vi "System Editor.vi"() -> ()   [LabVIEW 2013]
uses:
  <vilib>/Utility/miscctls.llb/LVBoundsTypeDef.ctl
  CRYCustom and Run Seq.llb/CRYCustom Cluster.ctl
  CRYCustom and Run Seq.llb/CRYProject Editor Global.vi
  CRYCustom and Run Seq.llb/CRYStepSetup Global.vi
  CRYCustom and Run Seq.llb/CRYMainGlobal.vi
  CRYCustom and Run Seq.llb/CRYMain Sub Window Global.vi
panel:
  out "Custom":string
  out "Custom Bk":string
  in  "AddStep":bool
  in  "Add Lib":bool
  in  "stop":bool
  in  "Load Test":bool
  out "EndFlag":bool
  out "Proper VI No":i32
  in  "Save As":bool
  in  "Load":bool
  in  "Revert":bool
  out "VIMiniumBound":T1
  in  "Board Tab":enum32{"Page 1"}(tab) caption="Control Tab"
  in  "Cancel":bool caption="Apply"
  in  "OK":bool caption="Apply"
  in  "Sub Board Tab":enum32{"Setting", "Help"}(tab)
  in  "Wait for completion":bool
  in  "Working Directory":path
  in  "Command Line":string
  in  "Help":string
  # "Reminder:  You must edit this custom step from\nwithin a sequence for it to remember your settings."
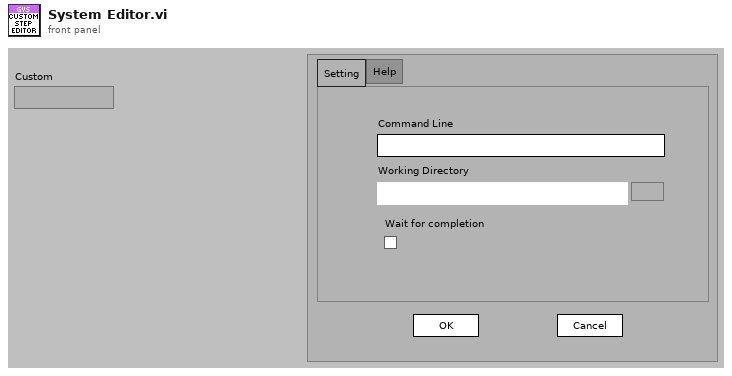
[diagram p1: front panel]
types:
  T1 = typedef "LVBoundsTypeDef.ctl" = cluster{"Width":u32, "Height":u32}
  T2 = cluster{"Command Line":string, "Working Directory":path, "Wait for completion":bool}
  T3 = typedef "CRYStep.ctl" = cluster{"No.VI":i32, "Category":string, "StepName":string, "Seq setup flattened":string, "Comment":string, "Steps config.":bool[], "Jump config":i32[], "Start":dbl, "Increment":dbl, "Name":string, "Unit":string, "Y data":u16, "Y prefix":string, "Y dB ref":dbl, "Y unit":string, "Repeat State Array":cluster{"Start":dbl, "Increment":dbl, "Count":i32, "Num":i32}[]}
  T4 = typedef "CRYCustom Cluster.ctl" = cluster{"Help":string, "Flatten Data":string}
  T5 = cluster{"Load Test":bool, "Add Lib":bool, "OK":bool, "Cancel":bool}
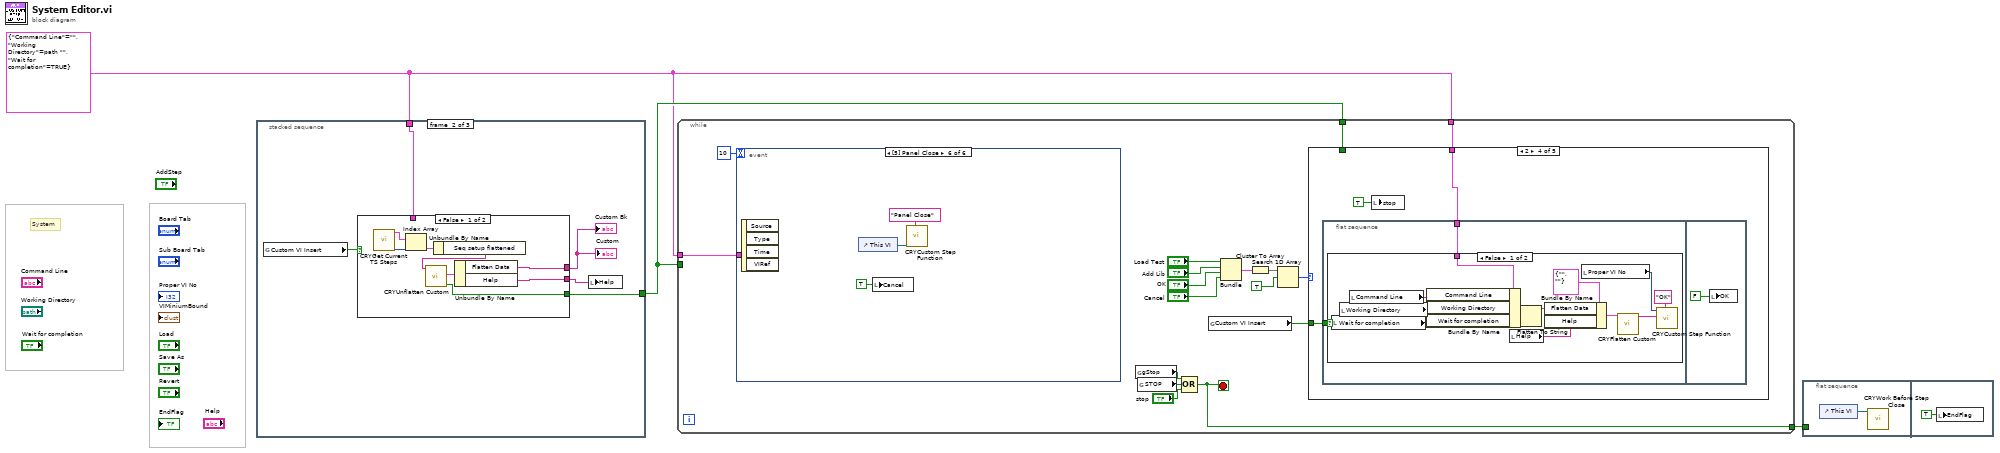
[diagram p0: block diagram]
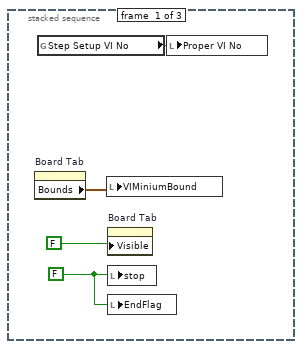
[diagram p2: hidden frame]
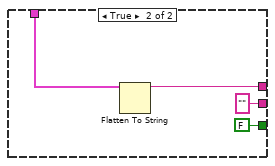
[diagram p3: hidden frame]
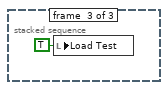
[diagram p4: hidden frame]
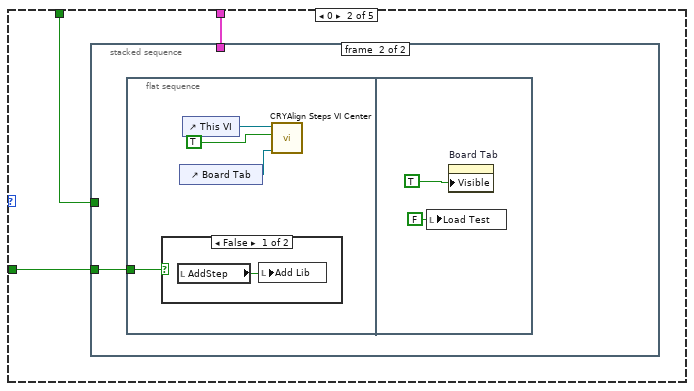
[diagram p6: hidden frame]
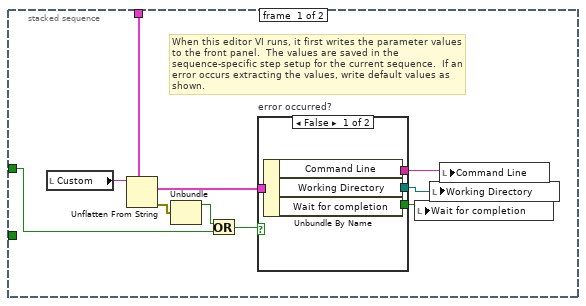
[diagram p7: hidden frame]
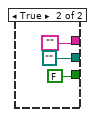
[diagram p8: hidden frame]
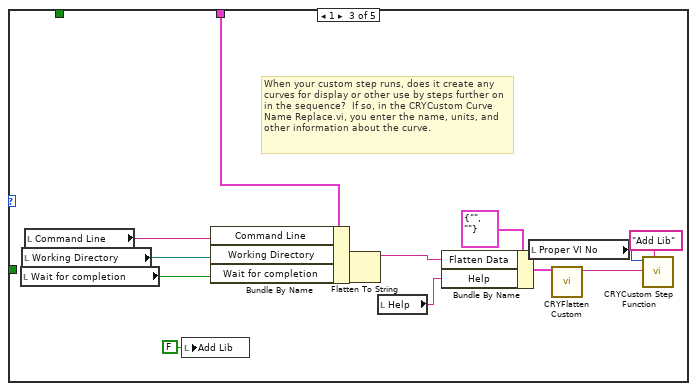
[diagram p10: hidden frame]
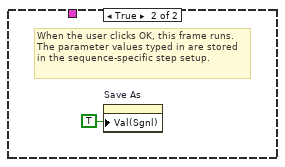
[diagram p11: hidden frame]
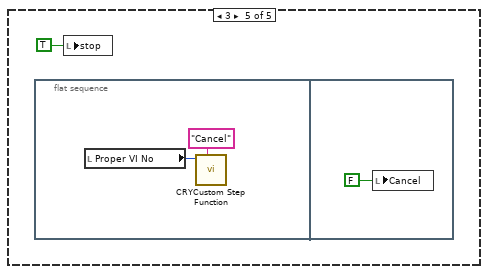
[diagram p12: hidden frame]
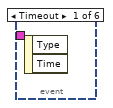
[diagram p13: hidden frame]
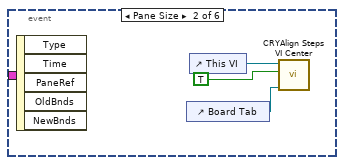
[diagram p14: hidden frame]
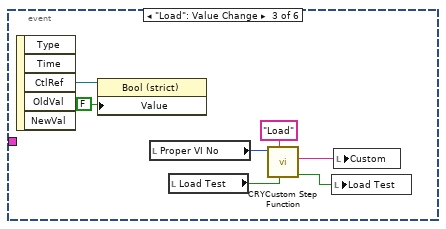
[diagram p15: hidden frame]
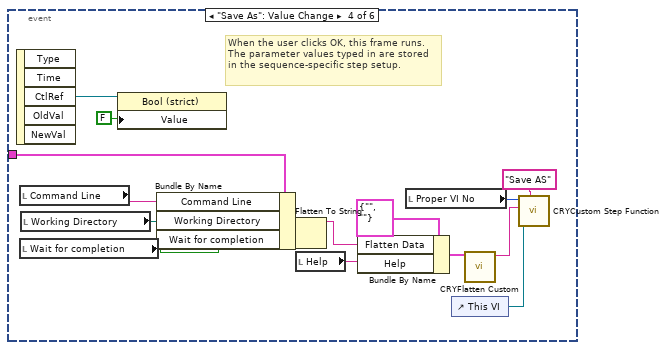
[diagram p16: hidden frame]
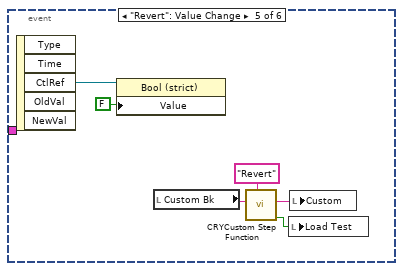
[diagram p17: hidden frame]
diagram:
  w1 = T2 {"Command Line"="", "Working Directory"=path "", "Wait for completion"=TRUE}
  # "System"
  n1 = stacked-sequence {
    tunnel: w1 -> [_ w11 _]
    tunnel: [_ w9 _] -> w2
    frame #0 {
      w4 = FALSE ("stop")
      n2 = property on="Board Tab" class="TabCtl (strict)"() -> ("Bounds"=w7:T1)  [unwired: 2 in, 2 out]
      n3 = global read "CRYProject Editor Global.vi" "Step Setup VI No"() -> (w5:i32)
      n4 = local write "VIMiniumBound"(w7) -> ()
      n5 = property on="Board Tab" class="TabCtl (strict)"("Visible"=FALSE ("Load Test")) -> ()  [unwired: 2 in, 2 out]
      n6 = local write "stop"(w4) -> ()
      n7 = local write "EndFlag"(w4) -> ()
      n8 = local write "Proper VI No"(w5) -> ()
    }
    frame #1 {
      n9 = global read "CRYStepSetup Global.vi" "Custom VI Insert"() -> (w12:bool)
      n10 = case shown="False" w12 {
        tunnel: [w14 w23] -> w8
        tunnel: w11 -> [_ w24]
        tunnel: [w16 FALSE ("Error?")] -> w9
        tunnel: [w13 "" ("Help")] -> w10
        frame False {
          n11 = call "CRYGet Current TS Steps.vi"() -> ("SelectStepNumber in Tree"=w18:i32, "Steps"=w19:T3[])  [unwired: 7 in, 3 out]
          n12 = Index Array(array=w19, index=w18) -> (element=w20:T3)
          n13 = Unbundle By Name(w20) -> ("Seq setup flattened"=w15:string)
          n14 = call "CRYUnflatten Custom.vi"("Unflatten Custom"=w15) -> ("Error?"=w16:bool, "Custom"=w17:T4)  [unwired: 8 in, 1 out]
          n15 = Unbundle By Name(w17) -> ("Flatten Data"=w14:string, "Help"=w13:string)
        }
        frame True {
          n16 = Flatten To String(anything=w24) -> (data string=w23:string)  [unwired: 1 in, 4 out]
        }
      }
      "Custom" <- w8
      "Custom Bk" <- w8
      n17 = local write "Help"(w10) -> ()
    }
    frame #2 {
      n18 = local write "Load Test"(TRUE ("Load Test")) -> ()
    }
  }
  n19 = while {
    tunnel: [w33] -> w3
    tunnel: w1 -> [w28]
    tunnel: w1 -> [w27]
    tunnel: w2 -> [w26]
    tunnel: w2 -> [_]
    stop <- w33 stop-if-true
    n20 = event shown="[5] Panel Close" {
      selector: _ -> [_ _ _ _ _ _]
      dyn-events: _ -> [_ _ _ _ _ _]
      timeout: 10 -> [_ _ _ _ _ _]
      tunnel: w27 -> [_ _ _ w128 _ _]
      event Timeout {
        n21 = event-data() -> ()  [unwired: 1 in, 2 out]
      }
      event Pane Size {
        n22 = event-data() -> ()  [unwired: 1 in, 5 out]
        n23 = control-ref of="Board Tab"() -> (w107:refnum<vi>)
        n24 = control-ref of="This VI"() -> (w108:refnum<vi>)
        n25 = call "CRYAlign Steps VI Center.vi"("Tab2"=w107, "Input/Output"=TRUE ("Preview"), "VIRef"=w108) -> ()  [unwired: 1 in, 8 out]
      }
      event "Load": Value Change {
        n26 = event-data() -> ("CtlRef"=w115:refnum<vi>)  [unwired: 1 in, 4 out]
        n27 = property class="Bool (strict)"(reference=w115, "Value"=FALSE) -> ()  [unwired: 1 in, 2 out]
        n28 = local read "Proper VI No"() -> (w113:i32)
        n29 = local read "Load Test"() -> (w110:bool)
        n30 = call "CRYCustom Step Function.vi"("bData"=w110, "sAction"="Load" ("Action"), "nData"=w113) -> ("bData Out"=w111:bool, "sData Out"=w112:string)  [unwired: 7 in]
        n31 = local write "Load Test"(w111) -> ()
        n32 = local write "Custom"(w112) -> ()
      }
      event "Save As": Value Change {
        # "When the user clicks OK, this frame runs.  The parameter values typed in are stored in the sequence-specific step setup."
        n33 = event-data() -> ("CtlRef"=w130:refnum<vi>)  [unwired: 1 in, 4 out]
        n34 = local read "Command Line"() -> (w127:string)
        n35 = local read "Wait for completion"() -> (w125:bool)
        n36 = local read "Working Directory"() -> (w126:path)
        n37 = property class="Bool (strict)"(reference=w130, "Value"=FALSE) -> ()  [unwired: 1 in, 2 out]
        n38 = Bundle By Name(cluster=w128, "Command Line"=w127, "Working Directory"=w126, "Wait for completion"=w125) -> (w129:T2)
        n39 = Flatten To String(anything=w129) -> (data string=w122:string)  [unwired: 1 in, 4 out]
        n40 = local read "Help"() -> (w121:string)
        n41 = Bundle By Name(cluster=T4 {"Help"="", "Flatten Data"=""} ("Custom"), "Flatten Data"=w122, "Help"=w121) -> (w123:T4)
        n42 = local read "Proper VI No"() -> (w118:i32)
        n43 = control-ref of="This VI"() -> (w119:refnum<vi>)
        n44 = call "CRYFlatten Custom.vi"("Custom"=w123) -> ("Flatten Custom String"=w117:string)  [unwired: 10 in]
        n45 = call "CRYCustom Step Function.vi"("sAction"="Save AS" ("Action"), "VI Ref"=w119, "sData"=w117, "nData"=w118) -> ()  [unwired: 6 in, 2 out]
      }
      event "Revert": Value Change {
        n46 = event-data() -> ("CtlRef"=w137:refnum<vi>)  [unwired: 1 in, 4 out]
        n47 = property class="Bool (strict)"(reference=w137, "Value"=FALSE) -> ()  [unwired: 1 in, 2 out]
        n48 = local read "Custom Bk"() -> (w134:string)
        n49 = call "CRYCustom Step Function.vi"("sAction"="Revert" ("Action"), "sData"=w134) -> ("bData Out"=w132:bool, "sData Out"=w133:string)  [unwired: 8 in]
        n50 = local write "Load Test"(w132) -> ()
        n51 = local write "Custom"(w133) -> ()
      }
      event Panel Close {
        n52 = event-data() -> ()  [unwired: 1 in, 4 out]
        n53 = control-ref of="This VI"() -> (w139:refnum<vi>)
        n54 = local write "Cancel"(TRUE ("Cancel")) -> ()
        n55 = call "CRYCustom Step Function.vi"("sAction"="Panel Close" ("Action"), "VI Ref"=w139) -> ()  [unwired: 8 in, 2 out]
      }
    }
    n56 = global read "CRYMain Sub Window Global.vi" "gStop"() -> (w36:bool)
    n57 = global read "CRYMainGlobal.vi" "STOP"() -> (w34:bool)
    n58 = Compound Arithmetic op=OR(w36, w34, "stop") -> (w33:bool)
    n59 = global read "CRYStepSetup Global.vi" "Custom VI Insert"() -> (w29:bool)
    n60 = Bundle("Load Test"="Load Test", "Add Lib"="Add Lib", "OK"="OK", "Cancel"="Cancel") -> (w40:T5)  [unwired: 1 out]
    n61 = Cluster To Array(cluster=w40) -> (array=w39:bool[])
    n62 = Search 1D Array(1D array=w39, element=TRUE) -> (index of element=w37:i32)  [unwired: 1 out]
    n63 = case shown="2" w37 {
      tunnel: w29 -> [_ w45 _ w85 _]
      tunnel: w28 -> [_ w44 w78 w84 _]
      tunnel: w26 -> [_ w43 _ _ _]
      frame Default {
      }
      frame 0 {
        n64 = stacked-sequence {
          tunnel: w45 -> [_ w63]
          tunnel: w44 -> [w51 _]
          tunnel: w43 -> [w46 _]
          frame #0 {
            # "When this editor VI runs, it first writes the parameter values to the front panel.  The values are saved in the sequence-specific step setup for the current sequence.  If an error occurs extracting the values, write default values as shown."
            n65 = local read "Custom"() -> (w47:string)
            n66 = Unflatten From String(type=w51, binary string=w47) -> (value=w54:T2, error out=w55:errorcluster)  [unwired: 1 in, 3 out]
            n67 = Unbundle(w55) -> ("status"=w52:bool)  [unwired: 2 out]
            n68 = Or(x=w52, y=w46) -> (x .or. y?=w53:bool)
            n69 = case "error occurred?" shown="False" w53 {
              tunnel: w54 -> [w59 _]
              tunnel: [w58 ""] -> w50
              tunnel: [w57 path ""] -> w49
              tunnel: [w56 FALSE ("Wait for completion")] -> w48
              frame False {
                n70 = Unbundle By Name(w59) -> ("Command Line"=w58:string, "Working Directory"=w57:path, "Wait for completion"=w56:bool)
              }
              frame True {
              }
            }
            n71 = local write "Wait for completion"(w48) -> ()
            n72 = local write "Working Directory"(w49) -> ()
            n73 = local write "Command Line"(w50) -> ()
          }
          frame #1 {
            n74 = flat-sequence {
              tunnel: w63 -> [w64]
              frame #0 {
                n75 = case shown="False" w64 {
                  frame False {
                    n76 = local read "AddStep"() -> (w68:bool)
                    n77 = local write "Add Lib"(w68) -> ()
                  }
                  frame True {
                  }
                }
                n78 = control-ref of="Board Tab"() -> (w65:refnum<vi>)
                n79 = control-ref of="This VI"() -> (w66:refnum<vi>)
                n80 = call "CRYAlign Steps VI Center.vi"("Tab2"=w65, "Input/Output"=TRUE ("Preview"), "VIRef"=w66) -> ()  [unwired: 1 in, 8 out]
              }
              frame #1 {
                n81 = local write "Load Test"(FALSE ("Load Test")) -> ()
                n82 = property on="Board Tab" class="TabCtl (strict)"("Visible"=TRUE ("Load Test")) -> ()  [unwired: 2 in, 2 out]
              }
            }
          }
        }
      }
      frame 1 {
        # "When your custom step runs, does it create any curves for display or other use by steps further on in the sequence?  If so, in the CRYCustom Curve Name Replace.vi, you enter the name, units, and other information about the curve."
        n83 = local read "Wait for completion"() -> (w82:bool)
        n84 = local read "Working Directory"() -> (w81:path)
        n85 = local read "Command Line"() -> (w80:string)
        n86 = local write "Add Lib"(FALSE ("Add Lib")) -> ()
        n87 = Bundle By Name(cluster=w78, "Command Line"=w80, "Working Directory"=w81, "Wait for completion"=w82) -> (w79:T2)
        n88 = Flatten To String(anything=w79) -> (data string=w76:string)  [unwired: 1 in, 4 out]
        n89 = local read "Help"() -> (w74:string)
        n90 = Bundle By Name(cluster=T4 {"Help"="", "Flatten Data"=""} ("Custom"), "Flatten Data"=w76, "Help"=w74) -> (w75:T4)
        n91 = local read "Proper VI No"() -> (w71:i32)
        n92 = call "CRYFlatten Custom.vi"("Custom"=w75) -> ("Flatten Custom String"=w72:string)  [unwired: 10 in]
        n93 = call "CRYCustom Step Function.vi"("sAction"="Add Lib" ("Action"), "sData"=w72, "nData"=w71) -> ()  [unwired: 7 in, 2 out]
      }
      frame 2 {
        n94 = flat-sequence {
          tunnel: w85 -> [w88]
          tunnel: w84 -> [w87]
          frame #0 {
            n95 = case shown="False" w88 {
              tunnel: w87 -> [w100 _]
              frame False {
                n96 = local read "Wait for completion"() -> (w96:bool)
                n97 = local read "Working Directory"() -> (w97:path)
                n98 = local read "Command Line"() -> (w98:string)
                n99 = Bundle By Name(cluster=w100, "Command Line"=w98, "Working Directory"=w97, "Wait for completion"=w96) -> (w99:T2)
                n100 = local read "Help"() -> (w93:string)
                n101 = Flatten To String(anything=w99) -> (data string=w94:string)  [unwired: 1 in, 4 out]
                n102 = Bundle By Name(cluster=T4 {"Help"="", "Flatten Data"=""} ("Custom"), "Flatten Data"=w94, "Help"=w93) -> (w92:T4)
                n103 = local read "Proper VI No"() -> (w90:i32)
                n104 = call "CRYFlatten Custom.vi"("Custom"=w92) -> ("Flatten Custom String"=w89:string)  [unwired: 10 in]
                n105 = call "CRYCustom Step Function.vi"("sAction"="OK" ("Action"), "sData"=w89, "nData"=w90) -> ()  [unwired: 7 in, 2 out]
              }
              frame True {
                # "When the user clicks OK, this frame runs.  The parameter values typed in are stored in the sequence-specific step setup."
                n106 = property on="Save As" class="Bool (strict)"("Val(Sgnl)"=TRUE ("Value (Signaling)")) -> ()  [unwired: 2 in, 2 out]
              }
            }
          }
          frame #1 {
            n107 = local write "OK"(FALSE ("OK")) -> ()
          }
        }
        n108 = local write "stop"(TRUE ("stop")) -> ()
      }
      frame 3 {
        n109 = flat-sequence {
          frame #0 {
            n110 = local read "Proper VI No"() -> (w105:i32)
            n111 = call "CRYCustom Step Function.vi"("sAction"="Cancel" ("Action"), "nData"=w105) -> ()  [unwired: 8 in, 2 out]
          }
          frame #1 {
            n112 = local write "Cancel"(FALSE ("Cancel")) -> ()
          }
        }
        n113 = local write "stop"(TRUE ("stop")) -> ()
      }
    }
  }
  n114 = flat-sequence {
    tunnel: w3 -> [_]
    frame #0 {
      n115 = control-ref of="This VI"() -> (w141:refnum<vi>)
      n116 = call "CRYWork Before Step Close.vi"("StepVI Ref"=w141) -> ()  [unwired: 11 in]
    }
    frame #1 {
      n117 = local write "EndFlag"(TRUE ("EndFlag")) -> ()
    }
  }
